vi "Plotter.vi"() -> ()   [LabVIEW 2021]
panel:
  out "Relay Supply Voltage":dbl[](graph)
  out "LabJack Supply Voltage":dbl[](graph)
  out "Solenoid Supply Voltage":dbl[](graph)
  out "LS2 Flowrate":dbl[](graph)
  out "LS1 Flowrate":dbl[](graph)
  out "LP1 Engine Thrust":dbl[](graph)
  out "PT3 Pressure":dbl[](graph)
  out "PT2 Pressure":dbl[](graph)
  out "PT1 Pressure":dbl[](graph)
  out "TC2 Temperature":dbl[](graph)
  out "TC1 Temperature":dbl[](graph)
  in  "?":bool
  in  "START/STOP DATA LOGGING":bool
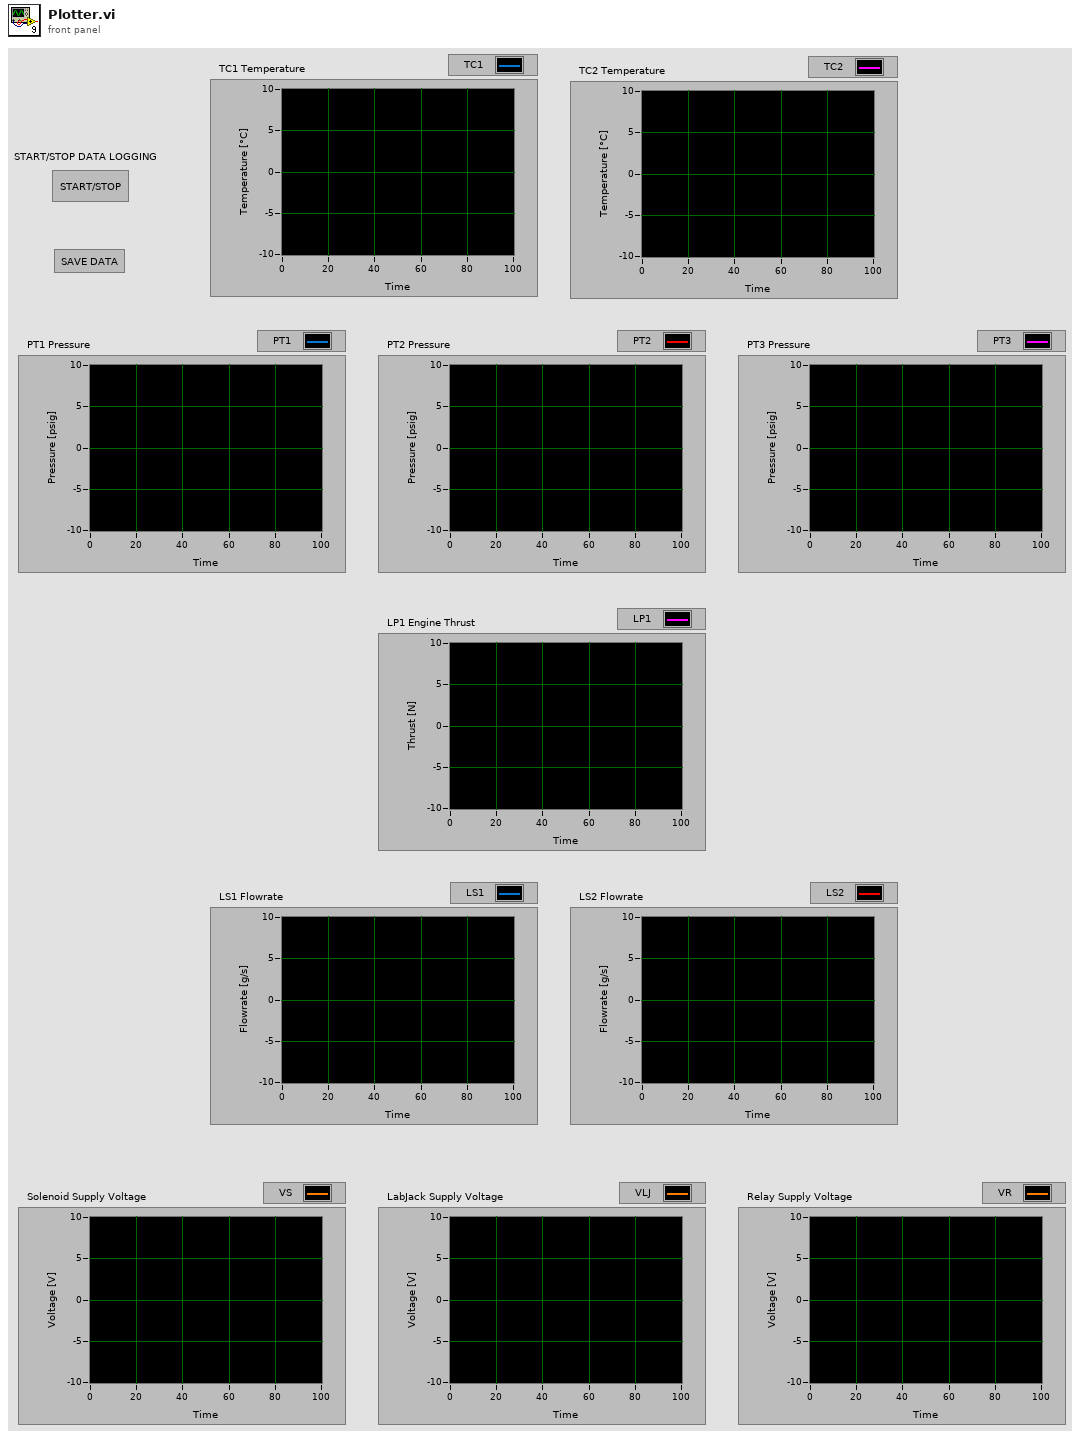
[diagram p1: front panel]
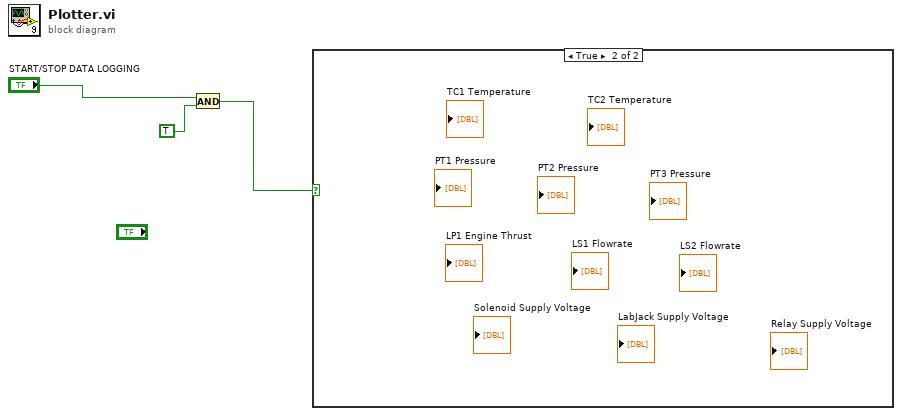
[diagram p0: block diagram]
diagram:
  n1 = And(x="START/STOP DATA LOGGING", y=TRUE) -> (x .and. y?=w1:bool)
  n2 = case shown="True" w1 {
    frame False {
    }
    frame True {
    }
  }
